vi "validate line configuration.vi"(7 "TDMS datalogger configuration":refnum<class "TDMS datalogger configuration.lvclass">, 11 "Mappings in":T1) -> (1 "valid?":bool, 2 "errors":string, 3 "Mappings out":T1)   [LabVIEW 2015, in "TDMS datalogger editor node.lvclass"]
uses:
  <vilib>/NI/DCAF/Modules/TDMSModule/editor/TDMS datalogger editor node.lvclass
  <vilib>/NI/Tag Bus Module Framework/channel/TBM channel.lvclass
  <vilib>/NI/DCAF/Modules/TDMSModule/module/configuration/TDMS datalogger configuration.lvclass
  <vilib>/NI/Tag Bus/tag/tag descriptor.lvclass/tag descriptor.ctl
  <vilib>/NI/Tag Bus/tag/read tag name.vi
  <vilib>/NI/Tag Bus/tag/read data type.vi
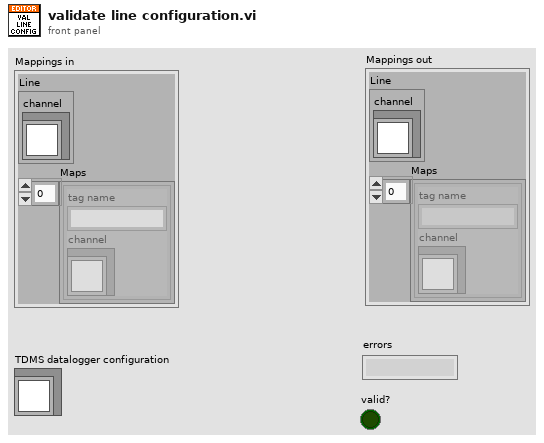
[diagram p1: front panel]
types:
  T1 = cluster{"Line":cluster{"channel":refnum<class "TBM channel.lvclass">}, "Maps":cluster{"tag name":string, "channel":refnum<class "TBM channel.lvclass">}[]}
  T2 = typedef "tag bus.lvlib/tag descriptor.lvclass/Data Type.ctl" = enum16{"Double", "Single", "I64", "I32", "I16", "I8", "U64", "U32", "U16", "U8", "Boolean", "String", "Array of Double", "Array of Single", "Array of I64", "Array of I32", "Array of I16", "Array of I8", "Array of U64", "Array of U32", "Array of U16", "Array of U8", "Array of Boolean", "Array of String"}
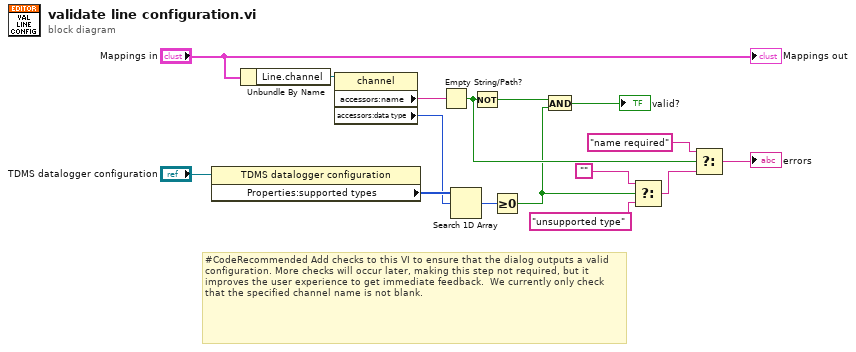
[diagram p0: block diagram]
diagram:
  # "#CodeRecommended Add checks to this VI to ensure that the dialog outputs a valid configuration. More checks will occur later, making this step not required, but it improves the user experience to get immediate feedback.  We currently only check that the specified channel name is not blank."
  n1 = property class="TDMS datalogger configuration"(reference="TDMS datalogger configuration") -> ("Properties:supported types"=w13:T2[])  [unwired: 1 in, 2 out]
  n2 = Unbundle By Name("Mappings in") -> ("Line.channel"=w16:refnum<class "TBM channel.lvclass">)
  n3 = property class="channel"(reference=w16) -> ("accessors:name"=w15:string, "accessors:data type"=w12:T2)  [unwired: 1 in, 2 out]
  n4 = Empty String/Path?(string/path=w15) -> (empty?=w9:bool)
  n5 = Search 1D Array(1D array=w13, element=w12) -> (index of element=w10:i32)  [unwired: 1 in]
  n6 = Not(x=w9) -> (.not. x?=w14:bool)
  n7 = Greater Or Equal To 0?(x=w10) -> (x >= 0?=w6:bool)
  n8 = And(x=w14, y=w6) -> (x .and. y?=→"valid?":bool)
  n9 = Select(t="", s=w6, f="unsupported type") -> (s? t:f=w4:string)
  n10 = Select(t="name required", s=w9, f=w4) -> (s? t:f=→"errors":string)
  "Mappings out" <- "Mappings in"
